vi "Read Pin.vi"(0 "Arduino in":refnum<class "Arduino.lvclass">, 5 "VISA resource name":refnum<visa-resource-name>, 9 "Port":dbl, 11 "error in (no error)":errorcluster) -> (4 "Arduino out":refnum<class "Arduino.lvclass">, 6 "VISA resource name 2":refnum<visa-resource-name>, 8 "Pin":bool, 10 "Response":string, 15 "error out":errorcluster)   [LabVIEW 2020, in "Arduino.lvclass"]
uses:
  Arduino.lvclass
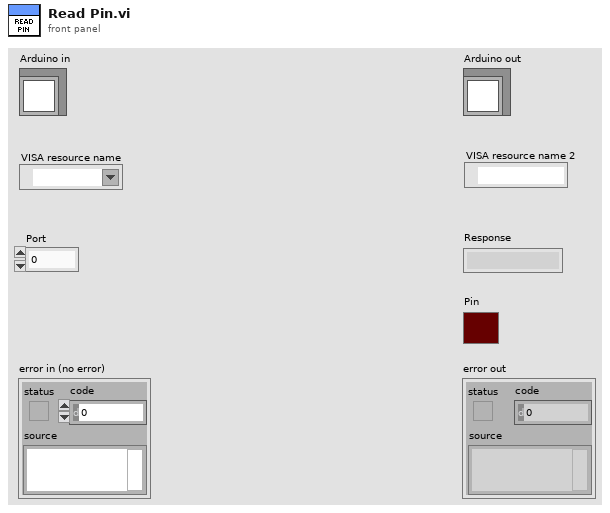
[diagram p1: front panel]
types:
  T1 = enum16{"Write", "Read", "Config", "Reset", "Close"}
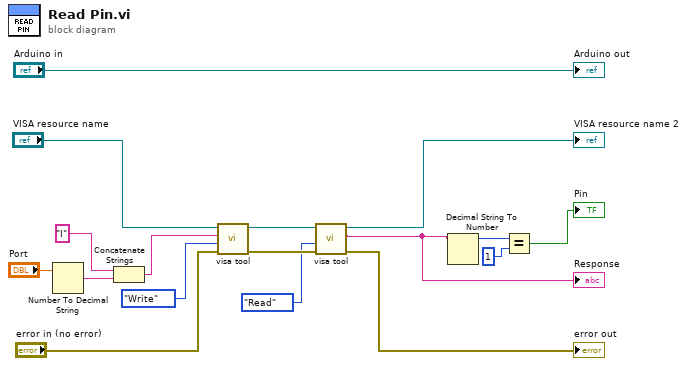
[diagram p0: block diagram]
diagram:
  n1 = Number To Decimal String(number="Port") -> (decimal integer string=w9:string)  [unwired: 1 in]
  n2 = Concatenate Strings("I" ("string"), w9) -> (w8:string)
  n3 = call "visa tool.vi"("error in (no error)"="error in (no error)", "Opciones"=T1."Write", "Write"=w8, "VISA com port"="VISA resource name") -> ("error out"=w5:errorcluster, "VISA com port 2"=w6:refnum<visa-resource-name>)  [unwired: 5 in, 1 out]
  n4 = call "visa tool.vi"("error in (no error)"=w5, "Opciones"=T1."Read", "VISA com port"=w6) -> ("error out"=→"error out":errorcluster, "Read"=w2:string, "VISA com port 2"=→"VISA resource name 2":refnum<visa-resource-name>)  [unwired: 6 in]
  "Response" <- w2
  n5 = Decimal String To Number(string=w2) -> (offset past number=w12:i32)  [unwired: 2 in, 1 out]
  n6 = Equal?(x=w12, y=1) -> (x = y?=→"Pin":bool)
  "Arduino out" <- "Arduino in"
